vi "test State Changes and Connections.vi"(8 "error in (no error)":errorcluster, 11 "TestCase in":refnum<class "SLSC Switch System Tests.lvclass">) -> (0 "error out":errorcluster, 3 "TestCase out":refnum<class "SLSC Switch System Tests.lvclass">)   [LabVIEW 2020, in "SLSC Switch System Tests.lvclass"]
uses:
  SLSC Switch System Tests.lvclass
  C:/Users/mjacobso/Desktop/SCM/niveristand-custom-device-testing-tools/VeriStandTestCase/VeriStandTestCase.lvclass
  SLSC Switch States.ctl
  SLSC Switch System Tests.lvclass/SLSC Switch System Tests.ctl
  <vilib>/NI VeriStand/Execution/Workspace/NI VeriStand - Set Single Channel Value.vi
  <vilib>/NI VeriStand/Execution/Workspace/NI_VS Workspace ExecutionAPI.lvlib
  <vilib>/addons/_JKI Toolkits/VI Tester/TestCase.llb/TestCase.lvclass
  C:/Program Files (x86)/National Instruments/LabVIEW 2020/vi.lib/addons/_JKI Toolkits/VI Tester/TestCase.llb/TestCase.lvclass
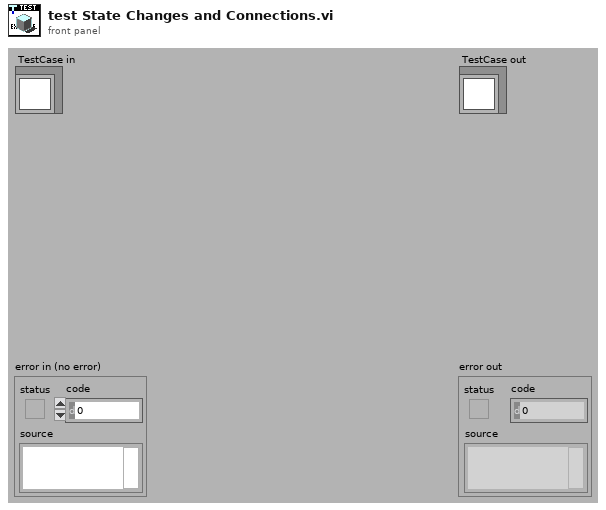
[diagram p1: front panel]
types:
  T1 = typedef "SLSC Switch System Tests.lvclass/SLSC Switch States.ctl" = cluster{"Channel Load States":cluster{"name":string, "value":i32}[], "Channel Bus States":cluster{"name":string, "value":i32}[], "Channel Pair States":cluster{"name":string, "value":i32}[]}
  T2 = typedef "NI_VS Workspace ExecutionAPI.lvlib/WorkspaceAPI.ctl" = refnum<k24>
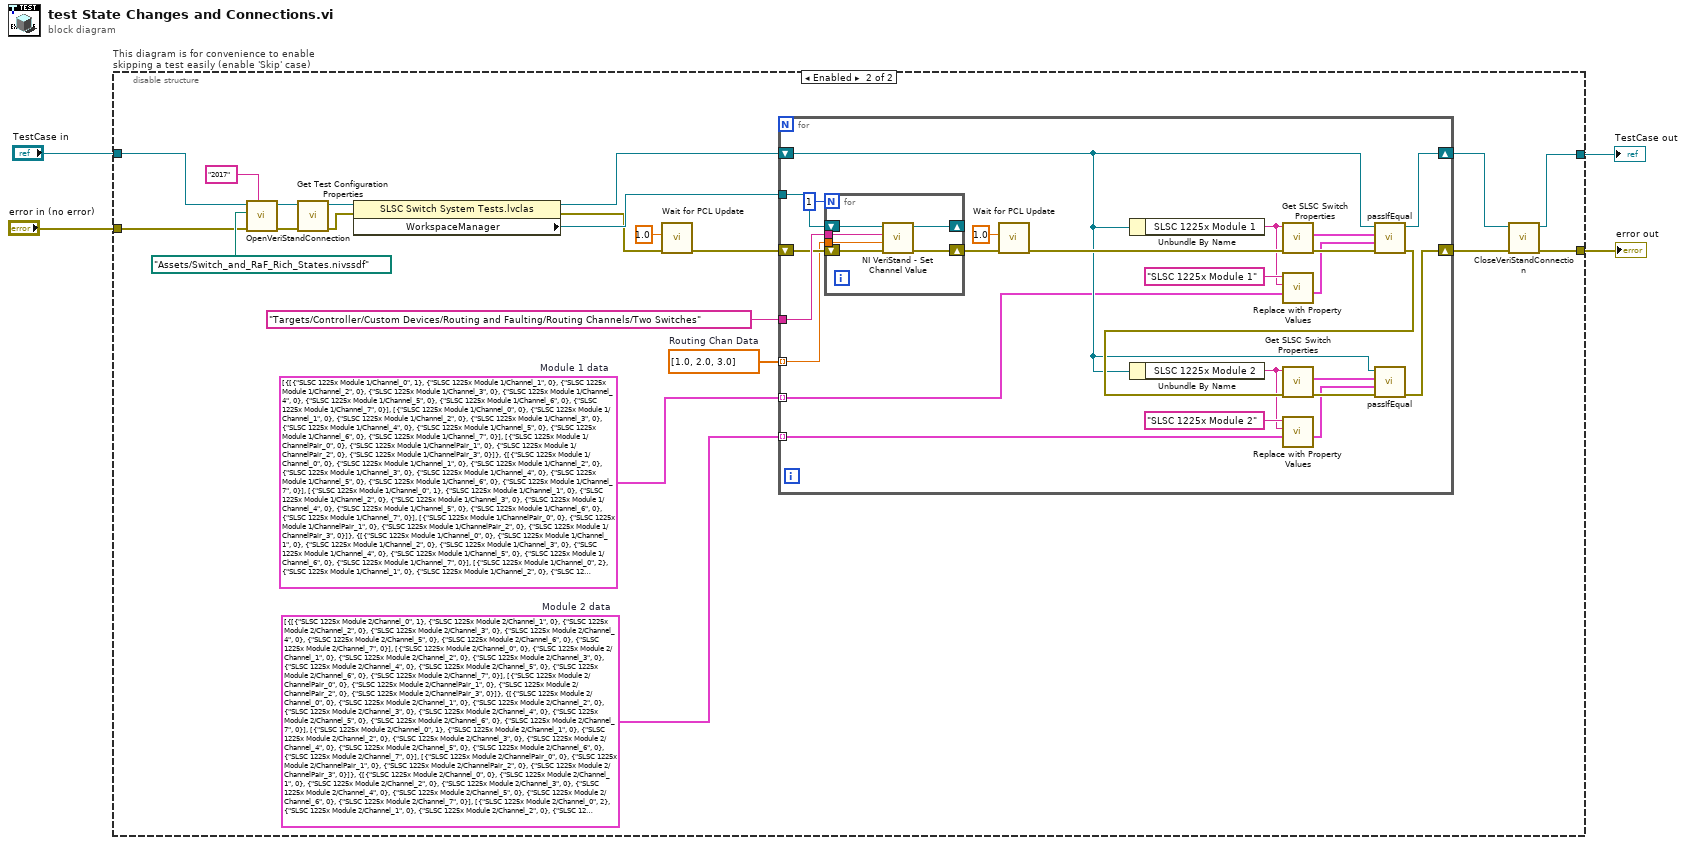
[diagram p0: block diagram]
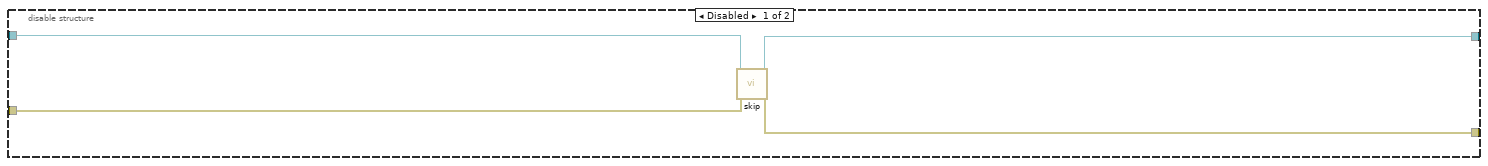
[diagram p2: hidden frame]
diagram:
  n1 = disable-structure "This diagram is for convenience to enable skipping a test easily (enable 'Skip' case)" shown="Enabled" {
    disable-tunnel: "TestCase in" -> [w8 w27]
    disable-tunnel: [w7 w22] -> w1
    disable-tunnel: [w6 w23] -> w3
    disable-tunnel: "error in (no error)" -> [w5 w26]
    frame Disabled {
      n2 = call <vilib>:"skip.vi"("error in (no error)"=w5, "TestCase in"=w8) -> ("error out"=w6:errorcluster, "TestCase out"=w7:refnum<class "SLSC Switch System Tests.lvclass">)  [unwired: 8 in]
    }
    frame Enabled {
      w10 = T1[] [{"Channel Load States"=[{"name"="SLSC 1225x Module 2/Channel_0", "value"=1}, {"name"="SLSC 1225x Module 2/Channel_1", "value"=0}, {"name"="SLSC 1225x Module 2/Channel_2", "value"=0}, {"name"="SLSC 1225x Module 2/Channel_3", "value"=0}, {"name"="SLSC 1225x Module 2/Channel_4", "value"=0}, {"name"="SLSC 1225x Module 2/Channel_5", "value"=0}, {"name"="SLSC 1225x Module 2/Channel_6", "value"=0}, {"name"="SLSC 1225x Module 2/Channel_7", "value"=0}], "Channel Bus States"=[{"name"="SLSC 1225x Module 2/Channel_0", "value"=0}, {"name"="SLSC 1225x Module 2/Channel_1", "value"=0}, {"name"="SLSC 1225x Module 2/Channel_2", "value"=0}, {"name"="SLSC 1225x Module 2/Channel_3", "value"=0}, {"name"="SLSC 1225x Module 2/Channel_4", "value"=0}, {"name"="SLSC 1225x Module 2/Channel_5", "value"=0}, {"name"="SLSC 1225x Module 2/Channel_6", "value"=0}, {"name"="SLSC 1225x Module 2/Channel_7", "value"=0}], "Channel Pair States"=[{"name"="SLSC 1225x Module 2/ChannelPair_0", "value"=0}, {"name"="SLSC 1225x Module 2/ChannelPair_1", "value"=0}, {"name"="SLSC 1225x Module 2/ChannelPair_2", "value"=0}, {"name"="SLSC 1225x Module 2/ChannelPair_3", "value"=0}]}, {"Channel Load States"=[{"name"="SLSC 1225x Module 2/Channel_0", "value"=0}, {"name"="SLSC 1225x Module 2/Channel_1", "value"=0}, {"name"="SLSC 1225x Module 2/Channel_2", "value"=0}, {"name"="SLSC 1225x Module 2/Channel_3", "value"=0}, {"name"="SLSC 1225x Module 2/Channel_4", "value"=0}, {"name"="SLSC 1225x Module 2/Channel_5", "value"=0}, {"name"="SLSC 1225x Module 2/Channel_6", "value"=0}, {"name"="SLSC 1225x Module 2/Channel_7", "value"=0}], "Channel Bus States"=[{"name"="SLSC 1225x Module 2/Channel_0", "value"=1}, {"name"="SLSC 1225x Module 2/Channel_1", "value"=0}, {"name"="SLSC 1225x Module 2/Channel_2", "value"=0}, {"name"="SLSC 1225x Module 2/Channel_3", "value"=0}, {"name"="SLSC 1225x Module 2/Channel_4", "value"=0}, {"name"="SLSC 1225x Module 2/Channel_5", "value"=0}, {"name"="SLSC 1225x Module 2/Channel_6", "value"=0}, {"name"="SLSC 1225x Module 2/Channel_7", "value"=0}], "Channel Pair States"=[{"name"="SLSC 1225x Module 2/ChannelPair_0", "value"=0}, {"name"="SLSC 1225x Module 2/ChannelPair_1", "value"=0}, {"name"="SLSC 1225x Module 2/ChannelPair_2", "value"=0}, {"name"="SLSC 1225x Module 2/ChannelPair_3", "value"=0}]}, {"Channel Load States"=[{"name"="SLSC 1225x Module 2/Channel_0", "value"=0}, {"name"="SLSC 1225x Module 2/Channel_1", "value"=0}, {"name"="SLSC 1225x Module 2/Channel_2", "value"=0}, {"name"="SLSC 1225x Module 2/Channel_3", "value"=0}, {"name"="SLSC 1225x Module 2/Channel_4", "value"=0}, {"name"="SLSC 1225x Module 2/Channel_5", "value"=0}, {"name"="SLSC 1225x Module 2/Channel_6", "value"=0}, {"name"="SLSC 1225x Module 2/Channel_7", "value"=0}], "Channel Bus States"=[{"name"="SLSC 1225x Module 2/Channel_0", "value"=2}, {"name"="SLSC 1225x Module 2/Channel_1", "value"=0}, {"name"="SLSC 1225x Module 2/Channel_2", "value"=0}, {"name"="SLSC 1225x Module 2/Channel_3", "value"=0}, {"name"="SLSC 1225x Module 2/Channel_4", "value"=0}, {"name"="SLSC 1225x Module 2/Channel_5", "value"=0}, {"name"="SLSC 1225x Module 2/Channel_6", "value"=0}, {"name"="SLSC 1225x Module 2/Channel_7", "value"=0}], "Channel Pair States"=[{"name"="SLSC 1225x Module 2/ChannelPair_0", "value"=0}, {"name"="SLSC 1225x Module 2/ChannelPair_1", "value"=0}, {"name"="SLSC 1225x Module 2/ChannelPair_2", "value"=0}, {"name"="SLSC 1225x Module 2/ChannelPair_3", "value"=0}]}]  # Module 2 data
      w9 = T1[] [{"Channel Load States"=[{"name"="SLSC 1225x Module 1/Channel_0", "value"=1}, {"name"="SLSC 1225x Module 1/Channel_1", "value"=0}, {"name"="SLSC 1225x Module 1/Channel_2", "value"=0}, {"name"="SLSC 1225x Module 1/Channel_3", "value"=0}, {"name"="SLSC 1225x Module 1/Channel_4", "value"=0}, {"name"="SLSC 1225x Module 1/Channel_5", "value"=0}, {"name"="SLSC 1225x Module 1/Channel_6", "value"=0}, {"name"="SLSC 1225x Module 1/Channel_7", "value"=0}], "Channel Bus States"=[{"name"="SLSC 1225x Module 1/Channel_0", "value"=0}, {"name"="SLSC 1225x Module 1/Channel_1", "value"=0}, {"name"="SLSC 1225x Module 1/Channel_2", "value"=0}, {"name"="SLSC 1225x Module 1/Channel_3", "value"=0}, {"name"="SLSC 1225x Module 1/Channel_4", "value"=0}, {"name"="SLSC 1225x Module 1/Channel_5", "value"=0}, {"name"="SLSC 1225x Module 1/Channel_6", "value"=0}, {"name"="SLSC 1225x Module 1/Channel_7", "value"=0}], "Channel Pair States"=[{"name"="SLSC 1225x Module 1/ChannelPair_0", "value"=0}, {"name"="SLSC 1225x Module 1/ChannelPair_1", "value"=0}, {"name"="SLSC 1225x Module 1/ChannelPair_2", "value"=0}, {"name"="SLSC 1225x Module 1/ChannelPair_3", "value"=0}]}, {"Channel Load States"=[{"name"="SLSC 1225x Module 1/Channel_0", "value"=0}, {"name"="SLSC 1225x Module 1/Channel_1", "value"=0}, {"name"="SLSC 1225x Module 1/Channel_2", "value"=0}, {"name"="SLSC 1225x Module 1/Channel_3", "value"=0}, {"name"="SLSC 1225x Module 1/Channel_4", "value"=0}, {"name"="SLSC 1225x Module 1/Channel_5", "value"=0}, {"name"="SLSC 1225x Module 1/Channel_6", "value"=0}, {"name"="SLSC 1225x Module 1/Channel_7", "value"=0}], "Channel Bus States"=[{"name"="SLSC 1225x Module 1/Channel_0", "value"=1}, {"name"="SLSC 1225x Module 1/Channel_1", "value"=0}, {"name"="SLSC 1225x Module 1/Channel_2", "value"=0}, {"name"="SLSC 1225x Module 1/Channel_3", "value"=0}, {"name"="SLSC 1225x Module 1/Channel_4", "value"=0}, {"name"="SLSC 1225x Module 1/Channel_5", "value"=0}, {"name"="SLSC 1225x Module 1/Channel_6", "value"=0}, {"name"="SLSC 1225x Module 1/Channel_7", "value"=0}], "Channel Pair States"=[{"name"="SLSC 1225x Module 1/ChannelPair_0", "value"=0}, {"name"="SLSC 1225x Module 1/ChannelPair_1", "value"=0}, {"name"="SLSC 1225x Module 1/ChannelPair_2", "value"=0}, {"name"="SLSC 1225x Module 1/ChannelPair_3", "value"=0}]}, {"Channel Load States"=[{"name"="SLSC 1225x Module 1/Channel_0", "value"=0}, {"name"="SLSC 1225x Module 1/Channel_1", "value"=0}, {"name"="SLSC 1225x Module 1/Channel_2", "value"=0}, {"name"="SLSC 1225x Module 1/Channel_3", "value"=0}, {"name"="SLSC 1225x Module 1/Channel_4", "value"=0}, {"name"="SLSC 1225x Module 1/Channel_5", "value"=0}, {"name"="SLSC 1225x Module 1/Channel_6", "value"=0}, {"name"="SLSC 1225x Module 1/Channel_7", "value"=0}], "Channel Bus States"=[{"name"="SLSC 1225x Module 1/Channel_0", "value"=2}, {"name"="SLSC 1225x Module 1/Channel_1", "value"=0}, {"name"="SLSC 1225x Module 1/Channel_2", "value"=0}, {"name"="SLSC 1225x Module 1/Channel_3", "value"=0}, {"name"="SLSC 1225x Module 1/Channel_4", "value"=0}, {"name"="SLSC 1225x Module 1/Channel_5", "value"=0}, {"name"="SLSC 1225x Module 1/Channel_6", "value"=0}, {"name"="SLSC 1225x Module 1/Channel_7", "value"=0}], "Channel Pair States"=[{"name"="SLSC 1225x Module 1/ChannelPair_0", "value"=0}, {"name"="SLSC 1225x Module 1/ChannelPair_1", "value"=0}, {"name"="SLSC 1225x Module 1/ChannelPair_2", "value"=0}, {"name"="SLSC 1225x Module 1/ChannelPair_3", "value"=0}]}]  # Module 1 data
      w17 = dbl[] [1.0, 2.0, 3.0]  # Routing Chan Data
      n3 = call-dynamic "OpenVeriStandConnection.vi"("Minimum VeriStand Version (2016)"="2017" ("Minimum VeriStand Version (2015)"), "error in (no error)"=w26, "System Definition File"=path "Assets/Switch_and_RaF_Rich_States.nivssdf", "VeriStand Test Case in"=w27) -> ("error out"=w24:errorcluster, "VeriStand Test Case out"=w12:refnum<class "SLSC Switch System Tests.lvclass">)  [unwired: 5 in, 1 out]
      n4 = call "Get Test Configuration Properties.vi"("error in (no error)"=w24, "Routing and Faulting System Tests in"=w12) -> ("error out"=w13:errorcluster, "Routing and Faulting System Tests out"=w11:refnum<class "SLSC Switch System Tests.lvclass">)  [unwired: 8 in]
      n5 = property class="SLSC Switch System Tests.lvclas"(reference=w11, error in=w13) -> (reference out=w20:refnum<class "SLSC Switch System Tests.lvclass">, error out=w15:errorcluster, "WorkspaceManager"=w21:T2)
      n6 = call "Wait for PCL Update"("error in (no error)"=w15, "Delay Time (s)"=1.0) -> ("error out"=w14:errorcluster)  [unwired: 9 in]
      n7 = for {
        tunnel: "Targets/Controller/Custom Devices/Routing and Faulting/Routing Channels/Two Switches" ("Channel") -> [w53]
        tunnel: w21 -> [w52]
        shift-right: [w39] -> w18
        shift-left: w14 -> [w51]
        shift-right: [w50] -> w19
        shift-left: w20 -> [w38]
        tunnel: w17 -> [w47] mode=indexing
        tunnel: w9 -> [w30] mode=indexing
        tunnel: w10 -> [w31] mode=indexing
        n8 = for {
          N: 1 -> [_]
          tunnel: w53 -> [w59]
          tunnel: w47 -> [w58]
          shift-right: [w54] -> _
          shift-left: w52 -> [w57]
          shift-right: [w55] -> w44
          shift-left: w51 -> [w56]
          n9 = call-poly <vilib>:"NI VeriStand - Set Channel Value.vi"("error in (no error)"=w56, "Value"=w58, "Channel"=w59, "WorkspaceManager in"=w57) -> ("error out"=w55:errorcluster, "WorkspaceManager out"=w54:T2)  [unwired: 6 in]
        }
        n10 = call "Wait for PCL Update"("error in (no error)"=w44, "Delay Time (s)"=1.0) -> ("error out"=w41:errorcluster)  [unwired: 9 in]
        n11 = Unbundle By Name(w38) -> ("SLSC 1225x Module 1"=w33:string)
        n12 = Unbundle By Name(w38) -> ("SLSC 1225x Module 2"=w32:string)
        n13 = call "Get SLSC Switch Properties.vi"("error in (no error)"=w41, "device"=w33) -> ("error out"=w49:errorcluster, "SLSC Switch States"=w46:T1)  [unwired: 8 in]
        n14 = call "Replace with Property Values.vi"("SLSC Switch States in"=w30, "replace string"=w33, "search string"="SLSC 1225x Module 1" ("name")) -> ("SLSC Switch States out"=w37:T1)  [unwired: 8 in]
        n15 = call "Replace with Property Values.vi"("SLSC Switch States in"=w31, "replace string"=w32, "search string"="SLSC 1225x Module 2" ("name")) -> ("SLSC Switch States out"=w36:T1)  [unwired: 8 in]
        n16 = call-dynamic "passIfEqual.vi"("error in (no error)"=w49, "y"=w37, "x"=w46, "TestCase in"=w38) -> ("error out"=w40:errorcluster, "TestCase out"=w50:refnum<class "SLSC Switch System Tests.lvclass">)  [unwired: 6 in]
        n17 = call "Get SLSC Switch Properties.vi"("error in (no error)"=w40, "device"=w32) -> ("error out"=w42:errorcluster, "SLSC Switch States"=w43:T1)  [unwired: 8 in]
        n18 = call-dynamic "passIfEqual.vi"("error in (no error)"=w42, "y"=w36, "x"=w43, "TestCase in"=w38) -> ("error out"=w39:errorcluster)  [unwired: 6 in, 1 out]
      }
      n19 = call-dynamic "CloseVeriStandConnection.vi"("error in (no error)"=w18, "VeriStand Test Case in"=w19) -> ("error out"=w23:errorcluster, "VeriStand Test Case out"=w22:refnum<class "SLSC Switch System Tests.lvclass">)  [unwired: 8 in]
    }
  }
  "error out" <- w3
  "TestCase out" <- w1
